vi "Test2_3c.vi"(7 "Report Enable":bool=TRUE, 8 "error in":errorcluster, 9 "Cycles Burst":i32=10000, 11 "Instrument VISA in":T1={"AWG VISA"="AGTMY51400121", "Oscilloscope  VISA "="labosc4", "Integration Board IP"="172.16.7.43", "connection ID"=refnum, "report out"=refnum, "report file path"=path "C:/CTA/LevelTriggerBoardTest/TestsData/sumtrigger_delay/tmp"}) -> (0 "error out":errorcluster, 3 "Instrument VISA out":T1={"AWG VISA"="AGTMY51400121", "Oscilloscope  VISA "="labosc4", "Integration Board IP"="172.16.7.43", "connection ID"=refnum, "report out"=refnum, "report file path"=path "C:/CTA/LevelTriggerBoardTest/TestsData/sumtrigger_delay/tmp"})   [LabVIEW 2009]
uses:
  <vilib>/Utility/NIReport.llb/NI_report.lvclass
  <vilib>/Utility/NIReport.llb/HTML/NI_HTML.lvclass
  <instrlib>/Agilent 8000 Series/Public/Configure/Configure Math (Binary Operation).vi
  <instrlib>/Agilent 81150/Agilent 81150.lvlib
  <instrlib>/Agilent 8000 Series/Agilent 8000 Series.lvlib
panel:
  in  "Vclip":i32[](array[numeric])
  in  "Array":dbl[](array[numeric])
  in  "attenuation":i32[](array[numeric])
  in  "channel":i32[](array[numeric])
  in  "Save NOW!":bool
  in  "End 2":bool=TRUE
  out "Data output":dbl[][](array[numeric])
  in  "sweep Vclip":T2={"MIN"=0.0, "MAX"=1200.0, "Steps"=25.0, "Log scale"=FALSE}
  out "Measurement":dbl=0.003283861386138614
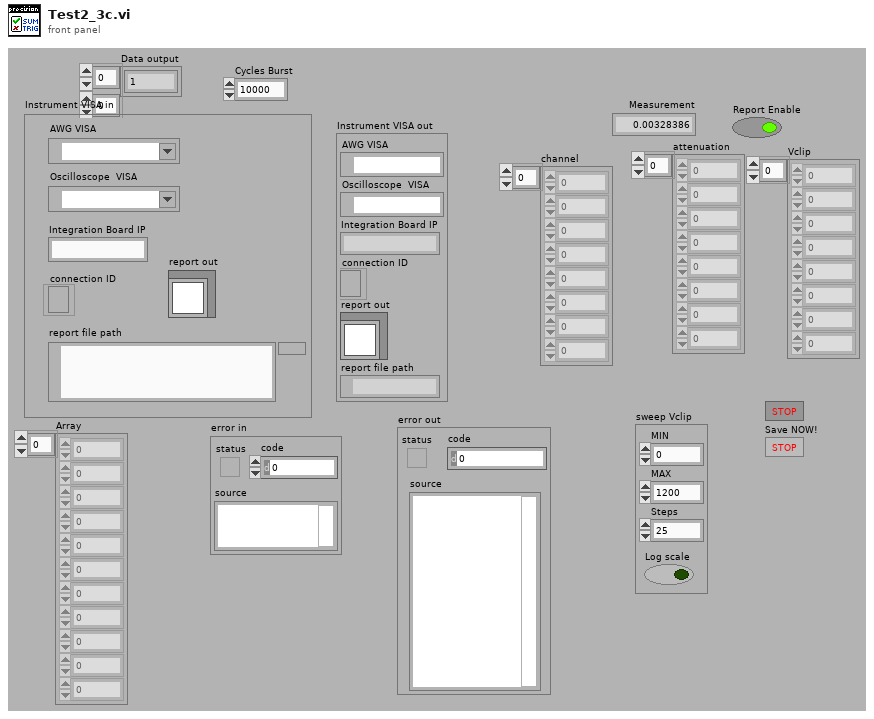
[diagram p1: front panel]
types:
  T1 = cluster{"AWG VISA":refnum<visa-resource-name>, "Oscilloscope  VISA ":refnum<visa-resource-name>, "Integration Board IP":string, "connection ID":refnum<k5>, "report out":refnum<class "NI_report.lvclass">, "report file path":path}
  T2 = cluster{"MIN":dbl, "MAX":dbl, "Steps":dbl, "Log scale":bool}
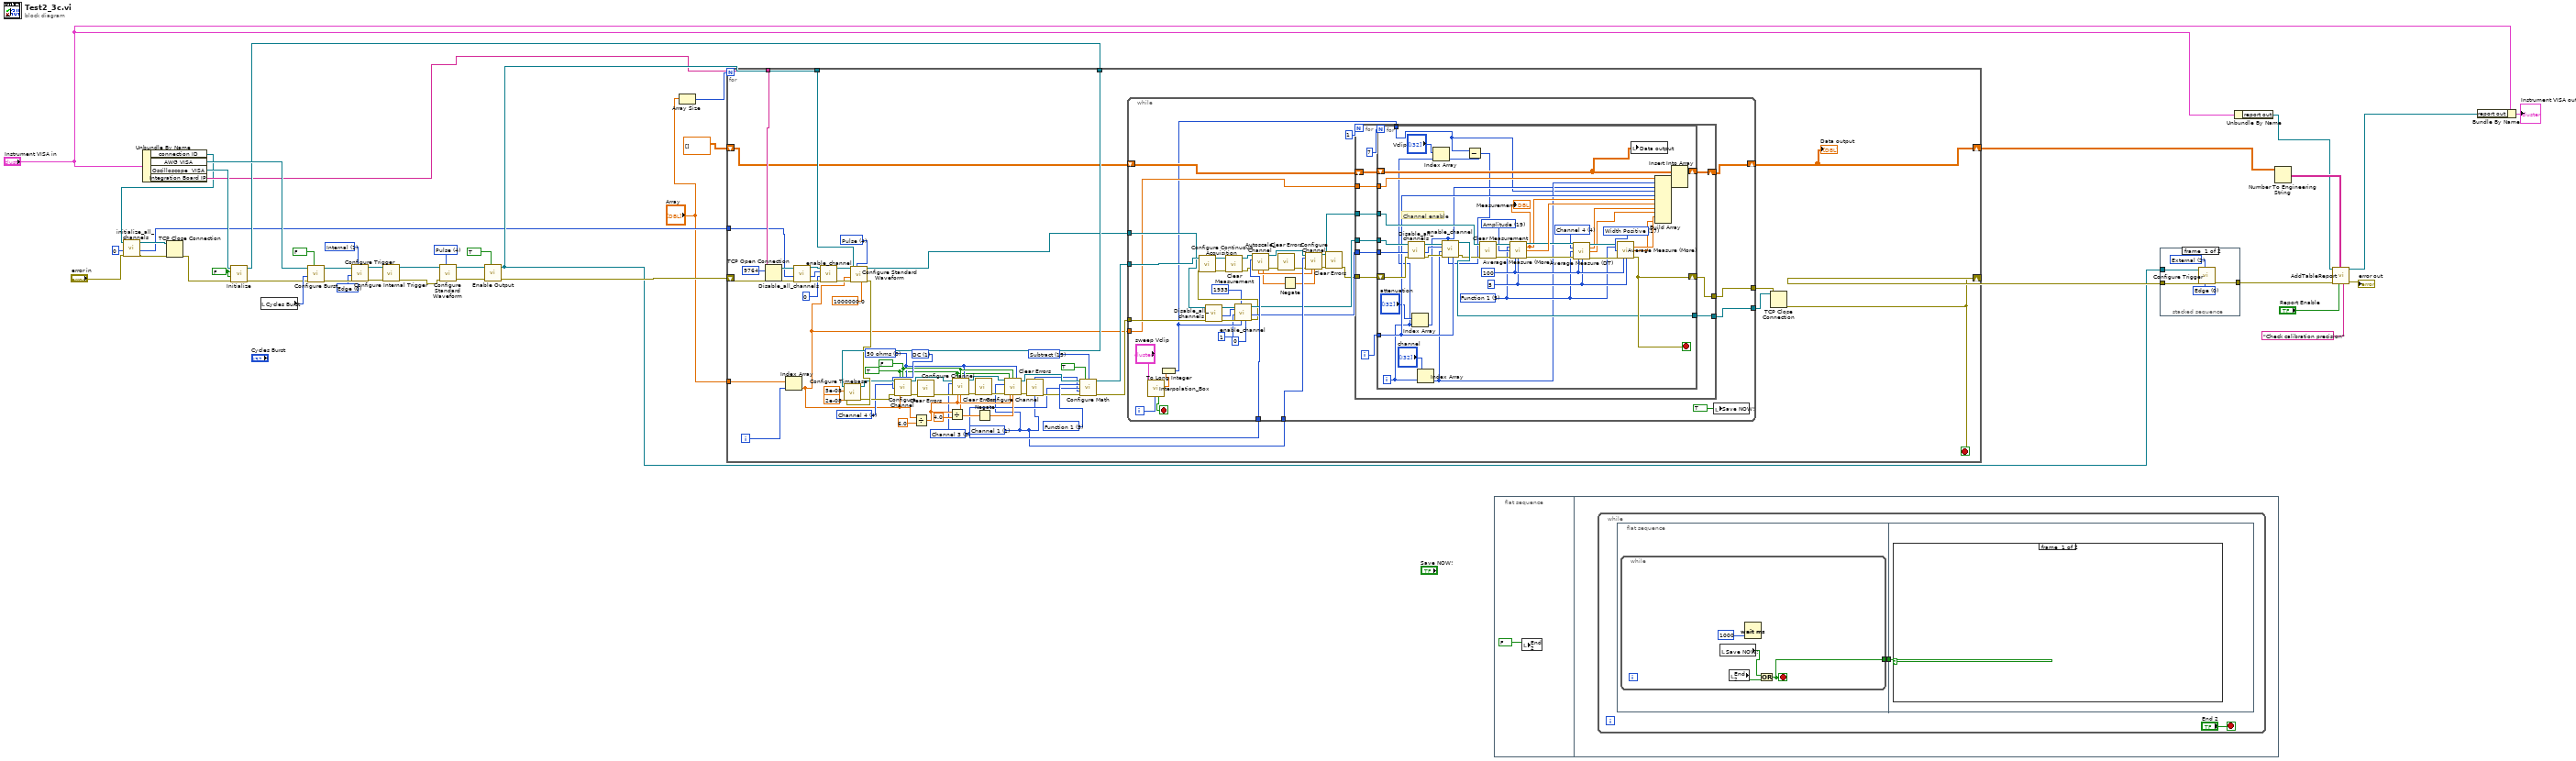
[diagram p0: block diagram]
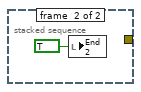
[diagram p2: hidden frame]
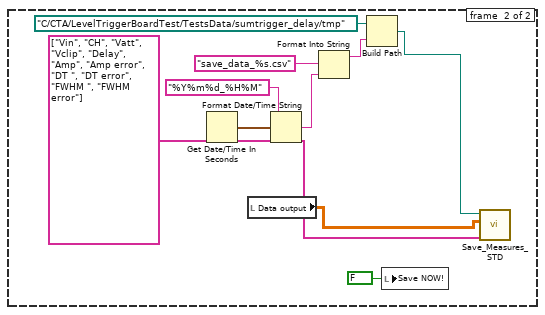
[diagram p3: hidden frame]
diagram:
  w25 = FALSE ("ID Query (True)")
  w32 = u16 1 items=["Immediate", "Internal", "External", "Software Trigger Function"] ("Trigger Source (0: Immediate)")
  w33 = u16 0 items=["Edge", "Level"] ("Trigger Mode (0: Edge)")
  w42 = u16 4 items=["Sine", "Square", "Ramp Up", "Ramp Down", "Pulse", "Noise", "DC"] ("Waveform (0: Sine)")
  n1 = Unbundle By Name("Instrument VISA in") -> ("connection ID"=w11:refnum<k5>, "AWG VISA"=w37:refnum<visa-resource-name>, "Oscilloscope  VISA"=w26:refnum<visa-resource-name>, "Integration Board IP"=w15:string)
  n2 = call "initialize_all_channels.vi"("error in"="error in", "id_in"=0, "connection ID"=w11) -> ("error out"=w13:errorcluster, "id_out"=w9:i32, "connection ID out"=w12:refnum<k5>)  [unwired: 6 in]
  n3 = TCP Close Connection(connection ID=w12, error in (no error)=w13) -> (error out=w18:errorcluster)  [unwired: 1 in, 1 out]
  n4 = call <instrlib>:"Initialize.vi"("error in (no error)"=w18, "Reset (True)"=w25, "ID Query (True)"=w25, "VISA resource name"=w26) -> ("error out"=w27:errorcluster, "VISA resource name out"=w16:refnum<visa-resource-name>)  [unwired: 6 in]
  n5 = local read "Cycles Burst"() -> (w38:i32)
  n6 = call <instrlib>:"Configure Burst.vi"("Enable Burst (F: Disable)"=FALSE, "error in (no error)"=w27, "Burst Count (2)"=w38, "VISA resource name"=w37) -> ("error out"=w35:errorcluster, "VISA resource name out"=w34:refnum<visa-resource-name>)  [unwired: 6 in]
  n7 = call <instrlib>:"Configure Trigger.vi"("Trigger Source (0: Immediate)"=w32, "error in (no error)"=w35, "Trigger Mode (0: Edge)"=w33, "VISA resource name"=w34) -> ("error out"=w31:errorcluster, "VISA resource name out"=w30:refnum<visa-resource-name>)  [unwired: 6 in]
  n8 = call <instrlib>:"Configure Internal Trigger.vi"("error in (no error)"=w31, "VISA resource name"=w30) -> ("error out"=w28:errorcluster, "VISA resource name out"=w29:refnum<visa-resource-name>)  [unwired: 8 in]
  n9 = call <instrlib>:"Configure Standard Waveform.vi"("Waveform (0: Sine)"=w42, "error in (no error)"=w28, "VISA resource name"=w29) -> ("error out"=w41:errorcluster, "VISA resource name out"=w40:refnum<visa-resource-name>)  [unwired: 7 in]
  n10 = call <instrlib>:"Enable Output.vi"("Enable Output (T: Enable)"=TRUE, "error in (no error)"=w41, "VISA resource name"=w40) -> ("error out"=w36:errorcluster, "VISA resource name out"=w17:refnum<visa-resource-name>)  [unwired: 7 in]
  n11 = Array Size(array="Array") -> (size(s)=w4:i32)
  n12 = for {
    N: w4 -> [_]
    shift-right: [w90] -> w24
    shift-left: w36 -> [w93]
    tunnel: w17 -> [w96]
    tunnel: w16 -> [w87]
    tunnel: w15 -> [w92]
    tunnel: w9 -> [w60]
    shift-right: [w45] -> w8
    shift-left: dbl[][] [] -> [w48]
    tunnel: "Array" -> [w44]
    i -> [w95]
    stop <- w90 stop-if-true
    w64 = TRUE ("Enable Channel (Enable)")
    w66 = FALSE ("BW Limit 20MHz (Disable)")
    w65 = u32 0 items=["50 ohms", "1 Mohms"] ("Input Impedance (1: 1 Mohms)")
    w76 = 4 items=["Channel 1"=1, "Channel 2"=2, "Channel 3"=3, "Channel 4"=4] ("Channel (1: Channel 1)")
    w77 = 1 items=["AC", "DC"] ("Vertical Coupling (1: DC)")
    w81 = u16 5 items=["Function 1"=5, "Function 2"=6, "Function 3"=7, "Function 4"=8] ("Math Channel (5: Function 1)")
    w82 = u16 15 items=["Add"=12, "Divide"=13, "Multiply"=14, "Subtract"=15, "Common Mode"=16, "Versus"=17] ("Math Operation (12: Add)")
    w47 = 3 items=["Channel 1"=1, "Channel 2"=2, "Channel 3"=3, "Channel 4"=4] ("Channel (1: Channel 1)")
    w46 = 1 items=["Channel 1"=1, "Channel 2"=2, "Channel 3"=3, "Channel 4"=4] ("Channel (1: Channel 1)")
    w97 = u16 4 items=["Sine", "Square", "Ramp Up", "Ramp Down", "Pulse", "Noise", "DC"] ("Waveform (0: Sine)")
    n13 = TCP Open Connection(address=w92, remote port or service name=u16 9764, error in (no error)=w93) -> (connection ID=w61:refnum<k5>, error out=w62:errorcluster)  [unwired: 2 in]
    n14 = Index Array(array=w44, index=w95) -> (element=w49:dbl)
    n15 = call "Disable_all_channels.vi"("error in"=w62, "id_in"=w60, "connection ID"=w61) -> ("error out"=w56:errorcluster, "id_out"=w55:i32, "connection ID out"=w58:refnum<k5>)  [unwired: 6 in]
    n16 = call "enable_channel.vi"("error in"=w56, "Channel"=u16 0 ("remote port or service name"), "id_in"=w55, "connection ID"=w58) -> ("error out"=w57:errorcluster, "connection ID out"=w59:refnum<k5>)  [unwired: 5 in, 1 out]
    n17 = call <instrlib>:"Configure Standard Waveform.vi"("Frequency (1000.0 Hz)"=1000000.0, "Waveform (0: Sine)"=w97, "error in (no error)"=w57, "Amplitude (1.0 Vpp)"=w49, "VISA resource name"=w96) -> ("error out"=w86:errorcluster)  [unwired: 5 in, 1 out]
    n18 = call <instrlib>:"Configure Timebase.vi"("error in (no error)"=w86, "Position (0.0 s)"=2e-08, "Timebase (0.005 s)"=5e-08, "VISA resource name"=w87) -> ("error out"=w78:errorcluster, "VISA resource name out"=w79:refnum<visa-resource-name>)  [unwired: 6 in]
    n19 = call <instrlib>:"Configure Channel.vi"("VISA resource name"=w79, "Enable Channel (Enable)"=w64, "BW Limit 20MHz (Disable)"=w66, "Input Impedance (1: 1 Mohms)"=w65, "Channel (1: Channel 1)"=w76, "Vertical Coupling (1: DC)"=w77, "error in (no error)"=w78, "Vertical Range (2.0 V)"=w49) -> ("VISA resource name out"=w74:refnum<visa-resource-name>, "error out"=w75:errorcluster)  [unwired: 6 in]
    n20 = Divide(x=w49, y=6.0) -> (x/y=w53:dbl)
    n21 = call <vilib>:"Clear Errors.vi"("error in (no error)"=w75) -> ("error out"=w71:errorcluster)  [unwired: 6 in]
    n22 = Divide(x=w53, y=4.0) -> (x/y=w50:dbl)
    n23 = call <instrlib>:"Configure Channel.vi"("VISA resource name"=w74, "Enable Channel (Enable)"=w64, "BW Limit 20MHz (Disable)"=w66, "Input Impedance (1: 1 Mohms)"=w65, "Channel (1: Channel 1)"=w47, "error in (no error)"=w71, "Vertical Range (2.0 V)"=w53, "Vertical Offset (0.0 V)"=w50) -> ("VISA resource name out"=w73:refnum<visa-resource-name>, "error out"=w70:errorcluster)  [unwired: 6 in]
    n24 = call <vilib>:"Clear Errors.vi"("error in (no error)"=w70) -> ("error out"=w69:errorcluster)  [unwired: 6 in]
    n25 = Negate(x=w50) -> (-x=w51:dbl)
    n26 = call <instrlib>:"Configure Channel.vi"("VISA resource name"=w73, "Enable Channel (Enable)"=w64, "BW Limit 20MHz (Disable)"=w66, "Input Impedance (1: 1 Mohms)"=w65, "Channel (1: Channel 1)"=w46, "error in (no error)"=w69, "Vertical Range (2.0 V)"=w53, "Vertical Offset (0.0 V)"=w51) -> ("VISA resource name out"=w72:refnum<visa-resource-name>, "error out"=w68:errorcluster)  [unwired: 6 in]
    n27 = call <vilib>:"Clear Errors.vi"("error in (no error)"=w68) -> ("error out"=w67:errorcluster)  [unwired: 6 in]
    n28 = call-poly <instrlib>:"Configure Math.vi"("VISA resource name"=w72, "Enable Math Channel (T:Enable)"=TRUE, "Math Operation (12: Add)"=w82, "Math Channel (5: Function 1)"=w81, "Math Operand (1: Channel 1)"=w47, "Math Operand (2: Channel 2)"=w46, "error in (no error)"=w67) -> ("VISA resource name out"=w85:refnum<visa-resource-name>, "error out"=w84:errorcluster)  [unwired: 7 in]
    n29 = while {
      tunnel: [w137] -> w91
      tunnel: [w136] -> w89
      tunnel: w85 -> [w135]
      tunnel: w84 -> [w134]
      tunnel: w59 -> [w133]
      tunnel: w49 -> [w132]
      shift-right: [w131] -> w45
      shift-left: w48 -> [w130]
      tunnel: w47 -> [w129]
      tunnel: w46 -> [w128]
      i -> [w126]
      stop <- w127 stop-if-true
      n30 = call "Interpolation_Box.vi"("Current step"=w126, "sweep parameters"="sweep Vclip") -> ("Value"=w124:dbl, "Finished"=w127:bool)  [unwired: 7 in, 1 out]
      n31 = To Long Integer(number=w124) -> (32bit integer=w125:i32)
      n32 = call "Disable_all_channels.vi"("error in"=w134, "connection ID"=w133) -> ("error out"=w122:errorcluster, "id_out"=w119:i32, "connection ID out"=w121:refnum<k5>)  [unwired: 7 in]
      n33 = call "enable_channel.vi"("Delay"=0, "V clip"=w125, "V att"=i16 1933 ("upper limit"), "error in"=w122, "Channel"=u32 1 ("Max Errors"), "id_in"=w119, "connection ID"=w121) -> ("error out"=w102:errorcluster, "id_out"=w117:i32, "connection ID out"=w120:refnum<k5>)  [unwired: 2 in]
      n34 = call <instrlib>:"Configure Continuous Acquisition.vi"("error in (no error)"=w102, "VISA resource name"=w135) -> ("error out"=w101:errorcluster, "VISA resource name out"=w103:refnum<visa-resource-name>)  [unwired: 8 in]
      n35 = call <instrlib>:"Clear Measurement.vi"("error in (no error)"=w101, "VISA resource name"=w103) -> ("error out"=w105:errorcluster, "VISA resource name out"=w104:refnum<visa-resource-name>)  [unwired: 8 in]
      n36 = call "Autoscale_Channel.vi"("error in"=w105, "Channel"=w129, "VISA resource name"=w104) -> ("error out"=w110:errorcluster, "VISA resource name out"=w115:refnum<visa-resource-name>, "Offset"=w108:dbl, "VerticalRange"=w114:dbl)  [unwired: 5 in]
      n37 = call <vilib>:"Clear Errors.vi"("error in (no error)"=w110) -> ("error out"=w111:errorcluster)  [unwired: 6 in]
      n38 = Negate(x=w108) -> (-x=w109:dbl)
      n39 = call <instrlib>:"Configure Channel.vi"("VISA resource name"=w115, "Channel (1: Channel 1)"=w128, "error in (no error)"=w111, "Vertical Range (2.0 V)"=w114, "Vertical Offset (0.0 V)"=w109) -> ("VISA resource name out"=w116:refnum<visa-resource-name>, "error out"=w112:errorcluster)  [unwired: 9 in]
      n40 = call <vilib>:"Clear Errors.vi"("error in (no error)"=w112) -> ("error out"=w113:errorcluster)  [unwired: 6 in]
      n41 = for {
        N: 1 -> [_]
        tunnel: [w148] -> w137
        tunnel: [w147] -> w136
        tunnel: w132 -> [w146]
        tunnel: w125 -> [w143]
        tunnel: w120 -> [w142]
        tunnel: w117 -> [w141]
        tunnel: w116 -> [w140]
        tunnel: w113 -> [w139]
        shift-right: [w145] -> w131
        shift-left: w130 -> [w144]
        i -> [w138]
        n42 = for {
          N: 7 -> [_]
          shift-right: [w191] -> w148
          shift-left: w139 -> [w187]
          tunnel: w142 -> [w188]
          tunnel: w140 -> [w184]
          tunnel: [w190] -> w147
          tunnel: w146 -> [w183]
          shift-right: [w181] -> w145
          shift-left: w144 -> [w159]
          tunnel: w143 -> [w151]
          tunnel: w141 -> [w161]
          tunnel: w138 -> [w160]
          i -> [w154]
          stop <- w191 stop-if-true
          w166 = u32 100 ("Averages")
          w165 = u32 5 ("Max Errors")
          w176 = 17 items=["Rise Time", "Fall Time", "Frequency", "Period", "Voltage RMS(AC)", "Voltage RMS(DC)", "Voltage RMS (AC,cycle)", "Voltage RMS (DC,cycle)", "Voltage Max", "Voltage Min", "Voltage Middle", "Voltage Vpp", "Voltage High", "Voltage Low", "Voltage Average", "Voltage Average (cycle)", "Width Negative", "Width Positive", "Duty Cycle Positive", "Amplitude", "Overshoot", "Preshoot", "Voltage Base", "Voltage Upper", "Time Max", "Time Min", "Color Grade Crossing", "Color Grade Eye Width", "Color Grade Eye Height", "Color Grade Eye Q-Factory", "Color Grade Eye Duty Cycle Distortion(Percent)", "Color Grade Eye Duty Cycle Distortion(Time)", "Color Grade Eye Jitter(PP)", "Color Grade Eye Width(RMS)", "Cycle-cycle Duty Jitter(Rising)", "Cycle-cycle Duty Jitter(Falling)", "Cycle-cycle Jitter(Rising)", "Cycle-cycle Jitter(Falling)", "Cycle-cycle - Width", "Cycle-cycle + Width", "Date Rate", "Unit Interval", "FFT Delta Frequency", "FFT Delta Magnitude", "FFT Frequency", "FFT Magnitude", "Slew Rate", "Area (Entire Display)", "Area(Single Cycle)", "Duty Cycle (Rising)", "Duty Cycle (Falling)"] ("Measurement Function (0: Rise Time)")
          w164 = u16 4 items=["Channel 1"=1, "Channel 2"=2, "Channel 3"=3, "Channel 4"=4, "Function 1"=5, "Function 2"=6, "Function 3"=7, "Function 4"=8, "Memory 1"=9, "Memory 2"=10, "Memory 3"=11, "Memory 4"=12] ("Channel1 (1: Channel 1)")
          w163 = 5 items=["Channel 1"=1, "Channel 2"=2, "Channel 3"=3, "Channel 4"=4, "Function 1"=5, "Function 2"=6, "Function 3"=7, "Function 4"=8, "Memory 1"=9, "Memory 2"=10, "Memory 3"=11, "Memory 4"=12] ("aa")
          w177 = 19 items=["Rise Time", "Fall Time", "Frequency", "Period", "Voltage RMS(AC)", "Voltage RMS(DC)", "Voltage RMS (AC,cycle)", "Voltage RMS (DC,cycle)", "Voltage Max", "Voltage Min", "Voltage Middle", "Voltage Vpp", "Voltage High", "Voltage Low", "Voltage Average", "Voltage Average (cycle)", "Width Negative", "Width Positive", "Duty Cycle Positive", "Amplitude", "Overshoot", "Preshoot", "Voltage Base", "Voltage Upper", "Time Max", "Time Min", "Color Grade Crossing", "Color Grade Eye Width", "Color Grade Eye Height", "Color Grade Eye Q-Factory", "Color Grade Eye Duty Cycle Distortion(Percent)", "Color Grade Eye Duty Cycle Distortion(Time)", "Color Grade Eye Jitter(PP)", "Color Grade Eye Width(RMS)", "Cycle-cycle Duty Jitter(Rising)", "Cycle-cycle Duty Jitter(Falling)", "Cycle-cycle Jitter(Rising)", "Cycle-cycle Jitter(Falling)", "Cycle-cycle - Width", "Cycle-cycle + Width", "Date Rate", "Unit Interval", "FFT Delta Frequency", "FFT Delta Magnitude", "FFT Frequency", "FFT Magnitude", "Slew Rate", "Area (Entire Display)", "Area(Single Cycle)", "Duty Cycle (Rising)", "Duty Cycle (Falling)"] ("Measurement Function (0: Rise Time)")
          # "Channel enable"
          n43 = call "Disable_all_channels.vi"("error in"=w187, "id_in"=w161, "connection ID"=w188) -> ("error out"=w186:errorcluster, "id_out"=w185:i32, "connection ID out"=w189:refnum<k5>)  [unwired: 6 in]
          n44 = Index Array(array="attenuation", index=w154) -> (element=w155:i32)
          n45 = Index Array(array="channel", index=w154) -> (element=w156:i32)
          n46 = Index Array(array="Vclip", index=w154) -> (element=w152:i32)
          n47 = Subtract(x=w151, y=w152) -> (x-y=w150:i32)
          n48 = call "enable_channel.vi"("Delay"=w160, "V clip"=w150, "V att"=w155, "error in"=w186, "Channel"=w156, "id_in"=w185, "connection ID"=w189) -> ("error out"=w162:errorcluster, "connection ID out"=w190:refnum<k5>)  [unwired: 2 in, 1 out]
          n49 = call <instrlib>:"Clear Measurement.vi"("error in (no error)"=w162, "VISA resource name"=w184) -> ("error out"=w178:errorcluster, "VISA resource name out"=w179:refnum<visa-resource-name>)  [unwired: 8 in]
          n50 = call "Average Measure (More).vi"("VISA resource name"=w179, "Channel (1: Channel 1)"=w163, "Measurement Function (0: Rise Time)"=w177, "error in (no error)"=w178, "Averages"=w166, "Max Errors"=w165) -> ("VISA resource name out"=w175:refnum<visa-resource-name>, "Measure Average"=w167:dbl, "Measure Error"=w180:dbl, "error out"=w172:errorcluster)  [unwired: 6 in]
          "Measurement" <- w167
          n51 = call "Average Measure (DT).vi"("VISA resource name"=w175, "Channel1 (1: Channel 1)"=w164, "Channel2 (2: Channel 2)"=w163, "error in (no error)"=w172, "Averages"=w166, "Max Errors"=w165) -> ("VISA resource name out"=w174:refnum<visa-resource-name>, "Measure Average"=w171:dbl, "Measure Error"=w170:dbl, "error out"=w173:errorcluster)  [unwired: 6 in]
          n52 = call "Average Measure (More).vi"("VISA resource name"=w174, "Channel (1: Channel 1)"=w163, "Measurement Function (0: Rise Time)"=w176, "error in (no error)"=w173, "Averages"=w166, "Max Errors"=w165) -> ("Measure Average"=w169:dbl, "Measure Error"=w168:dbl, "error out"=w191:errorcluster)  [unwired: 6 in, 1 out]
          n53 = local write "Data output"(w159) -> ()
          n54 = Build Array(w183, w156, w155, w151, w160, w167, w180, w171, w170, w169, w168) -> (w182:dbl[])
          n55 = Insert Into Array(array=w159, new element=w182) -> (w181:dbl[][])  [unwired: 2 in]
        }
      }
      n56 = local write "Save NOW!"(TRUE ("Save NOW! 2")) -> ()
    }
    "Data output" <- w45
    n57 = TCP Close Connection(connection ID=w89, error in (no error)=w91) -> (error out=w90:errorcluster)  [unwired: 1 in, 1 out]
  }
  n58 = flat-sequence {
    frame #0 {
      n59 = local write "End 2"(FALSE ("End")) -> ()
    }
    frame #1 {
      n60 = while {
        stop <- "End 2" stop-if-true
        n61 = flat-sequence {
          tunnel: [w195] -> w193
          tunnel: w193 -> [w200]
          frame #0 {
            n62 = while {
              tunnel: [w196] -> w195
              stop <- w196 stop-if-true
              n63 = local read "Save NOW!"() -> (w197:bool)
              n64 = local read "End 2"() -> (w198:bool)
              n65 = Wait (ms)(milliseconds to wait=u32 1000) -> ()  [unwired: 1 out]
              n66 = Or(x=w197, y=w198) -> (x .or. y?=w196:bool)
            }
          }
          frame #1 {
            n67 = case shown="True" w200 {
              frame #0 {
              }
              frame #1 {
                n68 = Get Date/Time In Seconds() -> (seconds since 1Jan1904=w209:timestamp)
                n69 = local read "Data output"() -> (w202:dbl[][])
                n70 = Format Date/Time String(time format string (%c)="%Y%m%d_%H%M", seconds (now)=w209) -> (date/time string=w207:string)  [unwired: 1 in]
                n71 = Format Into String(format string="save_data_%s.csv", w207) -> (resulting string=w206:string)  [unwired: 2 in, 1 out]
                n72 = Build Path(base path=path "C:/CTA/LevelTriggerBoardTest/TestsData/sumtrigger_delay/tmp", name or relative path=w206) -> (appended path=w205:path)
                n73 = local write "Save NOW!"(FALSE ("Save NOW!")) -> ()
                n74 = call "Save_Measures_STD.vi"("appended array"=string[] ["Vin", "CH", "Vatt", "Vclip", "Delay", "Amp", "Amp error", "DT ", "DT error", "FWHM ", "FWHM error"], "Data in"=w202, "file path (dialog if empty)"=w205) -> ()  [unwired: 9 in]
              }
            }
          }
        }
      }
    }
  }
  n75 = stacked-sequence {
    tunnel: w24 -> [w213 _]
    tunnel: [w212 _] -> w20
    tunnel: w17 -> [w211 _]
    frame #0 {
      w214 = u16 2 items=["Immediate", "Internal", "External", "Software Trigger Function"] ("Trigger Source (0: Immediate)")
      w215 = u16 0 items=["Edge", "Level"] ("Trigger Mode (0: Edge)")
      n76 = call <instrlib>:"Configure Trigger.vi"("Trigger Source (0: Immediate)"=w214, "error in (no error)"=w213, "Trigger Mode (0: Edge)"=w215, "VISA resource name"=w211) -> ("error out"=w212:errorcluster)  [unwired: 6 in, 1 out]
    }
    frame #1 {
      n77 = local write "End 2"(TRUE ("End 2")) -> ()
    }
  }
  n78 = Unbundle By Name("Instrument VISA in") -> ("report out"=w5:refnum<class "NI_report.lvclass">)
  n79 = Number To Engineering String(4:w8) -> (0:w6:string[][])  [unwired: 3 in]
  n80 = call "AddTableReport.vi"("Table title"="Check calibration precision", "Report Enable"="Report Enable", "Data"=w6, "error in"=w20, "report in"=w5) -> ("error out"=→"error out":errorcluster, "report out"=w21:refnum<class "NI_report.lvclass">)  [unwired: 5 in]
  n81 = Bundle By Name(cluster="Instrument VISA in", "report out"=w21) -> (→"Instrument VISA out":T1)
